vi "PantherLAB_RemoveInstructionsBookmarks.vi"(9 "Ephemeral Scripting Info":T1, 10 "Event Info":T2 {"timeout (ms)" min=-1 step=1}, 11 "Module Info":T5) -> (0 "error out":errorcluster)   [LabVIEW 2016]
doc: "This is a scripting plugin that uses the same code to create controls and indicators to any node in the block diagram."
uses:
  <vilib>/Delacor/Delacor QMH/Libraries/_Scripting Support/Module Info--cluster.ctl
  <vilib>/Delacor/Delacor QMH/Libraries/_Scripting Support/Module Type--enum.ctl
  <vilib>/Delacor/Delacor QMH/Libraries/_Scripting Support/Event Info (New)--cluster.ctl
  <vilib>/Delacor/Delacor QMH/Libraries/_Scripting Support/Event Type (New)--enum.ctl
  <vilib>/Delacor/Delacor QMH/Libraries/_Scripting Support/Request Scoping--enum.ctl
  <vilib>/Delacor/Delacor QMH/Libraries/_Scripting Support/Ephemeral Scripting Info--cluster.ctl
  <vilib>/Utility/traverseref.llb/TRef TravTarget.ctl
  <resource>/dialog/lvconfig.llb/LV Config Read Boolean.vi
  <vilib>/Delacor/Delacor QMH/Libraries/_Scripting Support/dqmh_lib_DQMH Scripting Support.lvlib
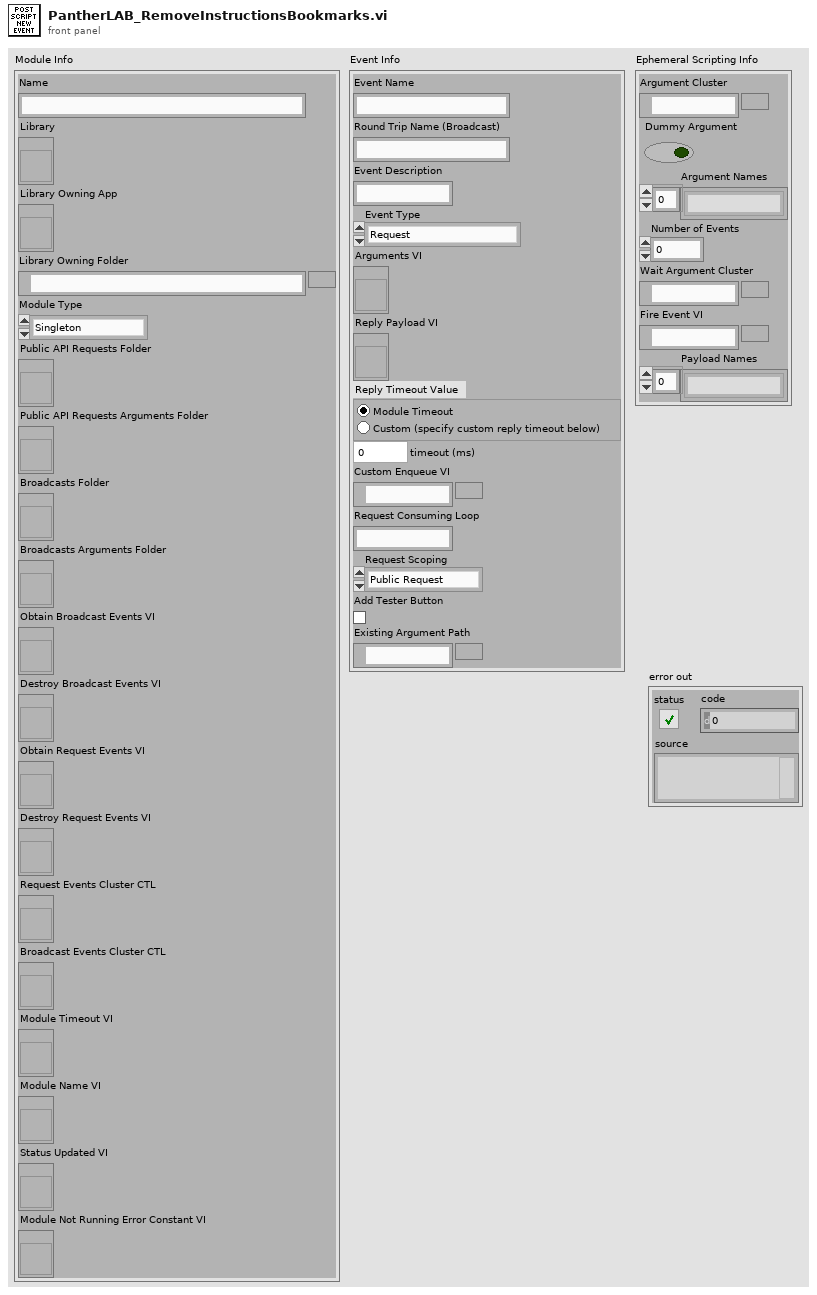
[diagram p1: front panel]
types:
  T1 = typedef "dqmh_lib_DQMH Scripting Support.lvlib/Ephemeral Scripting Info--cluster.ctl" = cluster{"Argument Cluster":path, "Dummy Argument":bool, "Argument Names":string[], "Number of Events":i32, "Wait Argument Cluster":path, "Fire Event VI":path, "Payload Names":string[]}
  T2 = typedef "dqmh_lib_DQMH Scripting Support.lvlib/Event Info (New)--cluster.ctl" = cluster{"Event Name":string, "Round Trip Name (Broadcast)":string, "Event Description":string, "Event Type":T3, "Arguments VI":refnum<vi>, "Reply Payload VI":refnum<vi>, "Reply Timeout Value":enum32{"Module Timeout", "Custom"}, "timeout (ms)":i32, "Custom Enqueue VI":path, "Request Consuming Loop":string, "Request Scoping":T4, "Add Tester Button":bool, "Existing Argument Path":path}
  T3 = typedef "dqmh_lib_DQMH Scripting Support.lvlib/Event Type (New)--enum.ctl" = enum16{"Request", "Broadcast", "Request and Wait for Reply", "Round Trip"}
  T4 = typedef "dqmh_lib_DQMH Scripting Support.lvlib/Request Scoping--enum.ctl" = enum16{"Public Request", "Private Request", "Local Instance"}
  T5 = typedef "dqmh_lib_DQMH Scripting Support.lvlib/Module Info--cluster.ctl" = cluster{"Name":string, "Library":refnum<vi>, "Library Owning App":refnum<vi>, "Library Owning Folder":path, "Module Type":T6, "Public API Requests Folder":refnum<vi>, "Public API Requests Arguments Folder":refnum<vi>, "Broadcasts Folder":refnum<vi>, "Broadcasts Arguments Folder":refnum<vi>, "Obtain Broadcast Events VI":refnum<vi>, "Destroy Broadcast Events VI":refnum<vi>, "Obtain Request Events VI":refnum<vi>, "Destroy Request Events VI":refnum<vi>, "Request Events Cluster CTL":refnum<vi>, "Broadcast Events Cluster CTL":refnum<vi>, "Module Timeout VI":refnum<vi>, "Module Name VI":refnum<vi>, "Status Updated VI":refnum<vi>, "Module Not Running Error Constant VI":refnum<vi>}
  T6 = typedef "dqmh_lib_DQMH Scripting Support.lvlib/Module Type--enum.ctl" = enum16{"Singleton", "Cloneable"}
  T7 = typedef "TRef TravTarget.ctl" = enum16{"FP", "BD", "Other"}
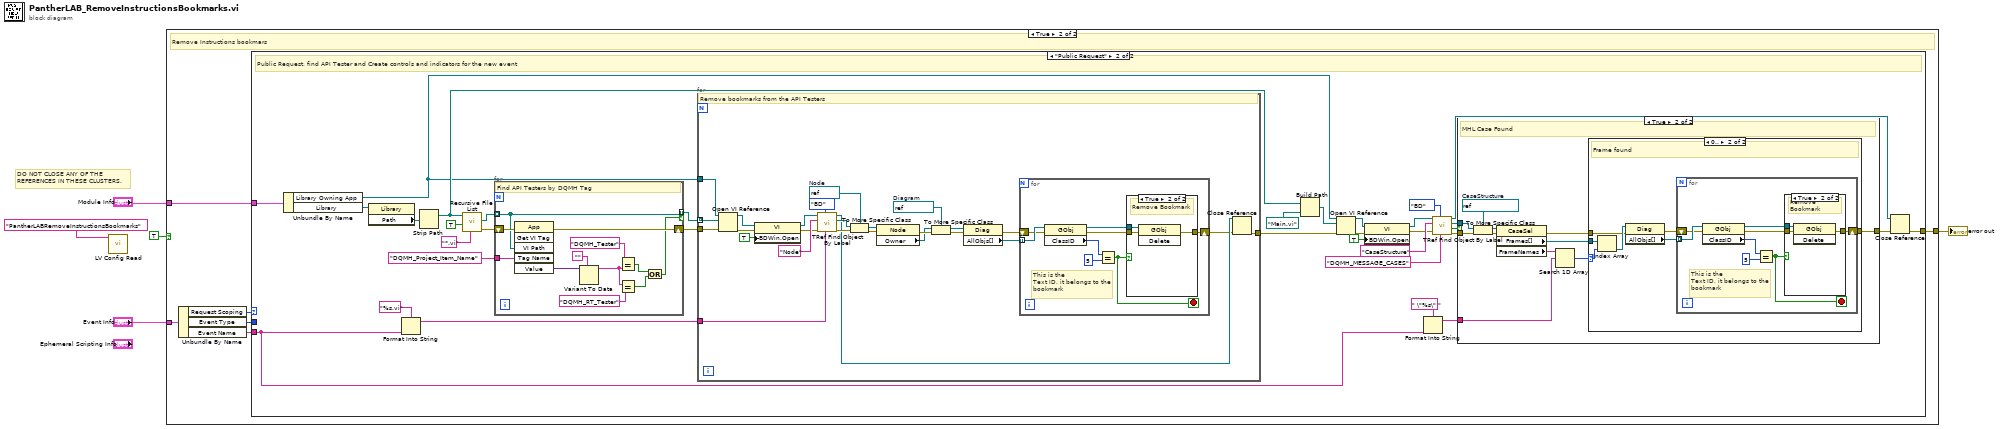
[diagram p0: block diagram]
diagram:
  # "DO NOT CLOSE ANY OF THE \nREFERENCES IN THESE CLUSTERS."
  n1 = call-poly <resource>:"LV Config Read.vi"("key"="PantherLABRemoveInstructionsBookmarks") -> ()  [unwired: 4 in, 3 out]
  n2 = case shown="True" TRUE {
    tunnel: "Module Info" -> [_ w11]
    tunnel: "Event Info" -> [_ w10]
    tunnel: [_ w6] -> w3
    frame False {
      # "Plugin Disabled"
    }
    frame True {
      # "Remove Instructions bookmars"
      n3 = Unbundle By Name(w10) -> ("Request Scoping"=w7:T4, "Event Type"=w8:T3, "Event Name"=w9:string)
      n4 = case shown="\"Public Request\"" w7 {
        tunnel: w11 -> [_ w45]
        tunnel: w9 -> [_ w18]
        tunnel: w8 -> [_ _]
        tunnel: [_ w21] -> w6
        frame "Private Request", Default {
          # "This plugin is suited for Public requests"
        }
        frame "Public Request" {
          # "Public Request, find API Tester and Create controls and indicators for the new event"
          n5 = Unbundle By Name(w45) -> ("Library Owning App"=w29:refnum<vi>, "Library"=w43:refnum<vi>)
          n6 = property class="Library"(reference=w43) -> ("Path"=w42:path)  [unwired: 1 in, 2 out]
          n7 = Format Into String(format string="%s.vi", w18) -> (resulting string=w33:string)  [unwired: 2 in, 1 out]
          n8 = Strip Path(path=w42) -> (stripped path=w32:path)  [unwired: 1 out]
          n9 = call <vilib>:"Recursive File List.vi"("pattern"="*.vi", "Continue Recursing on Error? (F)"=TRUE, "Folder Path"=w32) -> ("error out"=w38:errorcluster, "All Files in Dir"=w39:path[])  [unwired: 4 in, 3 out]
          n10 = for {
            tunnel: w39 -> [w79] mode=indexing
            shift-right: [w85] -> w36
            shift-left: w38 -> [w89]
            tunnel: "DQMH_Project_Item_Name" -> [w88]
            tunnel: [w79] -> w35 mode=indexing if=w78
            # "Find API Testers by DQMH Tag"
            n11 = invoke class="App" method="Get VI Tag"(error in=w89, "VI Path"=w79, "Tag Name"=w88) -> (error out=w85:errorcluster, "Value"=w87:variant)  [unwired: 3 in, 4 out]
            n12 = Variant To Data(type="", Variant=w87) -> (data=w82:string)  [unwired: 1 in, 1 out]
            n13 = Equal?(x="DQMH_Tester", y=w82) -> (x = y?=w81:bool)
            n14 = Equal?(x=w82, y="DQMH_RT_Tester" ("x")) -> (x = y?=w80:bool)
            n15 = Or(x=w81, y=w80) -> (x .or. y?=w78:bool)
          }
          n16 = for {
            tunnel: w36 -> [w115]
            tunnel: w35 -> [w114] mode=indexing
            tunnel: w29 -> [w113]
            tunnel: w33 -> [w106]
            tunnel: [w103] -> w44
            w94 = refnum<vi> refnum  # Diagram
            w107 = refnum<vi> refnum  # Node
            # "Remove bookmarks from the API Testers"
            n17 = Open VI Reference(application reference (local)=w113, vi path=w114, error in (no error)=w115) -> (vi reference=w100:refnum<vi>, error out=w112:errorcluster)  [unwired: 3 in]
            n18 = property class="VI"(reference=w100, error in=w112, "BDWin.Open"=TRUE ("Block Diagram Window:Open")) -> (reference out=w99:refnum<vi>, error out=w101:errorcluster)
            n19 = call <vilib>:"TRef Find Object By Label.vi"("Label"=w106, "Traverse Target"=TRef_TravTarget."BD", "error in (no error)"=w101, "Class Name"="Node", "VI Ref"=w99) -> ("error out"=w109:errorcluster, "Found Obj Ref"=w108:refnum<vi>, "dup VI Ref"=w102:refnum<vi>)  [unwired: 3 in, 1 out]
            n20 = To More Specific Class(target class=w107, reference=w108, error in=w109) -> (specific class reference=w105:refnum<vi>, error out=w104:errorcluster)
            n21 = property class="Node"(reference=w105, error in=w104) -> (error out=w97:errorcluster, "Owner"=w95:refnum<vi>)  [unwired: 1 out]
            n22 = To More Specific Class(target class=w94, reference=w95, error in=w97) -> (specific class reference=w93:refnum<vi>, error out=w96:errorcluster)
            n23 = property class="Diag"(reference=w93, error in=w96) -> (error out=w91:errorcluster, "AllObjs[]"=w92:refnum<vi>[])  [unwired: 1 out]
            n24 = for {
              tunnel: w92 -> [w123] mode=indexing
              shift-right: [w116] -> w90
              shift-left: w91 -> [w119]
              stop <- w120 stop-if-true
              # "This is the\nText ID, it belongs to the\nbookmark"
              n25 = property class="GObj"(reference=w123, error in=w119) -> (reference out=w117:refnum<vi>, error out=w118:errorcluster, "ClassID"=w122:u32)
              n26 = Equal?(x=w122, y=u32 5) -> (x = y?=w120:bool)
              n27 = case shown="True" w120 {
                tunnel: w118 -> [w124 w126]
                tunnel: w117 -> [_ w127]
                tunnel: [w124 w125] -> w116
                frame False {
                }
                frame True {
                  # "Remove Bookmark"
                  n28 = invoke class="GObj" method="Delete"(reference=w127, error in=w126) -> (error out=w125:errorcluster)  [unwired: 1 in, 2 out]
                }
              }
            }
            n29 = Close Reference(reference=w102, error in (no error)=w90) -> (error out=w103:errorcluster)
          }
          n30 = Build Path(base path=w32, name or relative path=path "Main.vi") -> (appended path=w30:path)
          n31 = Open VI Reference(application reference (local)=w29, vi path=w30, error in (no error)=w44) -> (vi reference=w15:refnum<vi>, error out=w16:errorcluster)  [unwired: 3 in]
          n32 = property class="VI"(reference=w15, error in=w16, "BDWin.Open"=TRUE ("Block Diagram Window:Open")) -> (reference out=w14:refnum<vi>, error out=w13:errorcluster)
          n33 = Format Into String(format string=" \"%s\" ", w18) -> (resulting string=w20:string)  [unwired: 2 in, 1 out]
          n34 = call <vilib>:"TRef Find Object By Label.vi"("Label"="DQMH_MESSAGE_CASES", "Traverse Target"=TRef_TravTarget."BD", "error in (no error)"=w13, "Class Name"="CaseStructure", "VI Ref"=w14) -> ("error out"=w26:errorcluster, "Found?"=w12:bool, "Found Obj Ref"=w25:refnum<vi>, "dup VI Ref"=w23:refnum<vi>)  [unwired: 3 in]
          n35 = case shown="True" w12 {
            tunnel: w26 -> [w46 w57]
            tunnel: w25 -> [_ w55]
            tunnel: [w46 w49] -> w22
            tunnel: w20 -> [_ w48]
            frame False {
            }
            frame True {
              w54 = refnum<vi> refnum  # CaseStructure
              # "MHL Case Found"
              n36 = To More Specific Class(target class=w54, reference=w55, error in=w57) -> (specific class reference=w53:refnum<vi>, error out=w56:errorcluster)
              n37 = property class="CaseSel"(reference=w53, error in=w56) -> (error out=w50:errorcluster, "Frames[]"=w52:refnum<vi>[], "FrameNames"=w47:string[])  [unwired: 1 out]
              n38 = Search 1D Array(1D array=w47, element=w48) -> (index of element=w51:i32)  [unwired: 1 in]
              n39 = case shown="0.." w51 {
                selector: w51 -> [_ w64]
                tunnel: w52 -> [_ w65]
                tunnel: w50 -> [w58 w60]
                tunnel: [w58 w59] -> w49
                frame Default {
                }
                frame 0.. {
                  # "Frame found"
                  n40 = Index Array(array=w65, index=w64) -> (element=w61:refnum<vi>)
                  n41 = property class="Diag"(reference=w61, error in=w60) -> (error out=w62:errorcluster, "AllObjs[]"=w63:refnum<vi>[])  [unwired: 1 out]
                  n42 = for {
                    tunnel: w63 -> [w73] mode=indexing
                    shift-right: [w66] -> w59
                    shift-left: w62 -> [w69]
                    stop <- w70 stop-if-true
                    # "This is the\nText ID, it belongs to the\nbookmark"
                    n43 = property class="GObj"(reference=w73, error in=w69) -> (reference out=w67:refnum<vi>, error out=w68:errorcluster, "ClassID"=w72:u32)
                    n44 = Equal?(x=w72, y=u32 5) -> (x = y?=w70:bool)
                    n45 = case shown="True" w70 {
                      tunnel: w68 -> [w74 w76]
                      tunnel: w67 -> [_ w77]
                      tunnel: [w74 w75] -> w66
                      frame False {
                      }
                      frame True {
                        # "Remove Bookmark"
                        n46 = invoke class="GObj" method="Delete"(reference=w77, error in=w76) -> (error out=w75:errorcluster)  [unwired: 1 in, 2 out]
                      }
                    }
                  }
                }
              }
            }
          }
          n47 = Close Reference(reference=w23, error in (no error)=w22) -> (error out=w21:errorcluster)
        }
      }
    }
  }
  "error out" <- w3
